vi "Status Alarm Condition.vi"(0 "VISA resource name":refnum<visa-resource-name>, 7 "Input (0: A)":u16(ring) items=["A", "B", "C", "D"], 11 "error in (no error)":errorcluster) -> (4 "VISA resource name out":refnum<visa-resource-name>, 8 "Alarm High Status":bool, 10 "Alarm Low Status":bool, 15 "error out":errorcluster)   [LabVIEW 2019, in "Lake Shore Cryotronics 340.lvlib"]
doc: "This VI indicates the status of the alarm for the selected input."
uses:
  Lake Shore Cryotronics 340.lvlib
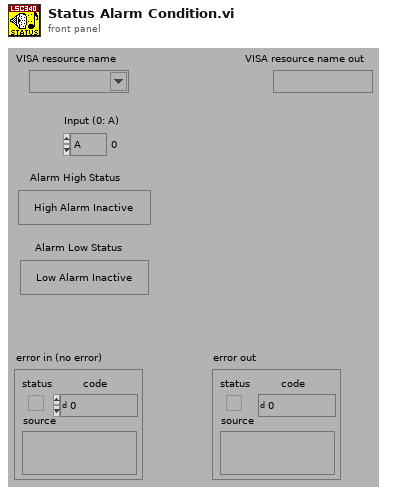
[diagram p1: front panel]
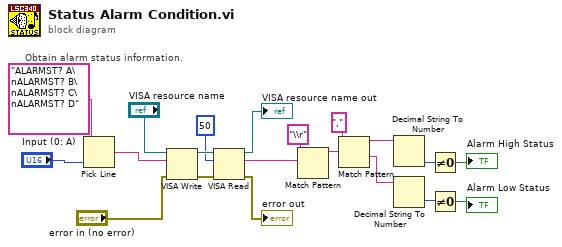
[diagram p0: block diagram]
diagram:
  # "Obtain alarm status information."
  n1 = Pick Line(multi-line string="ALARMST? A\nALARMST? B\nALARMST? C\nALARMST? D", line index="Input (0: A)") -> (output string=w1:string)  [unwired: 1 in]
  n2 = VISA Write(VISA resource name="VISA resource name", write buffer=w1, error in (no error)="error in (no error)") -> (VISA resource name out=w18:refnum<visa-resource-name>, error out=w17:errorcluster)  [unwired: 1 out]
  n3 = VISA Read(VISA resource name=w18, byte count=50, error in (no error)=w17) -> (VISA resource name out=→"VISA resource name out":refnum<visa-resource-name>, read buffer=w15:string, error out=→"error out":errorcluster)  [unwired: 1 out]
  n4 = Match Pattern(string=w15, regular expression="\\r") -> (before substring=w12:string)  [unwired: 1 in, 3 out]
  n5 = Match Pattern(string=w12, regular expression=",") -> (before substring=w11:string, after substring=w10:string)  [unwired: 1 in, 2 out]
  n6 = Decimal String To Number(string=w11) -> (number=w9:i32)  [unwired: 2 in, 1 out]
  n7 = Decimal String To Number(string=w10) -> (number=w8:i32)  [unwired: 2 in, 1 out]
  n8 = Not Equal To 0?(x=w9) -> (x != 0?=→"Alarm High Status":bool)
  n9 = Not Equal To 0?(x=w8) -> (x != 0?=→"Alarm Low Status":bool)
